vi "Motion Plot sub_VI.vi"(8 "Motion Parameters":T1={"Decel Time (s)"=0.0, "Accel Time (s)"=0.0, "Total Time (s)"=0.0, "Max Accel (mm/s^2)"=0.0, "Max Decel (mm/s^2)"=0.0, "Time step (s)"=0.01} {"Time step (s)" min=0.001}) -> (1 "Acceleration":dbl[](graph), 2 "Velocity":dbl[](graph), 3 "Displacement":dbl[](graph), 4 "V max (mm/s)":dbl, 5 "Dist max (mm)":dbl)   [LabVIEW 2017]
panel:
  # "Use 0.01s"
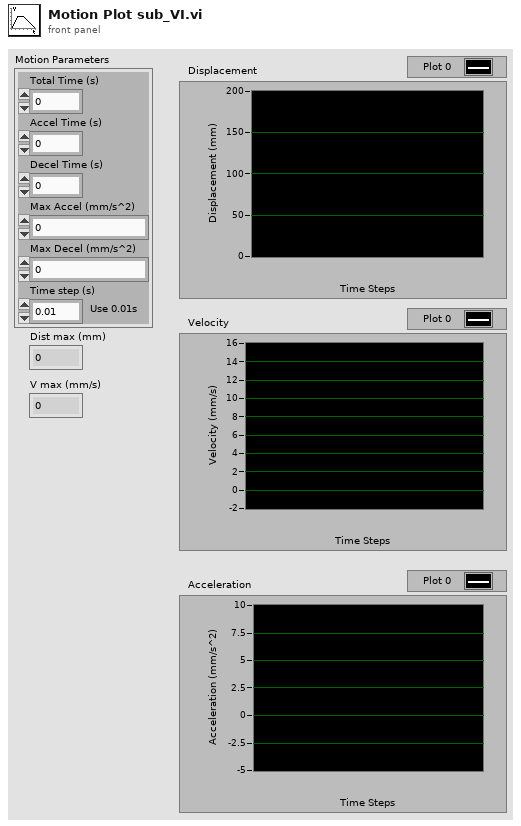
[diagram p1: front panel]
types:
  T1 = cluster{"Decel Time (s)":dbl, "Accel Time (s)":dbl, "Total Time (s)":dbl, "Max Accel (mm/s^2)":dbl, "Max Decel (mm/s^2)":dbl, "Time step (s)":dbl}
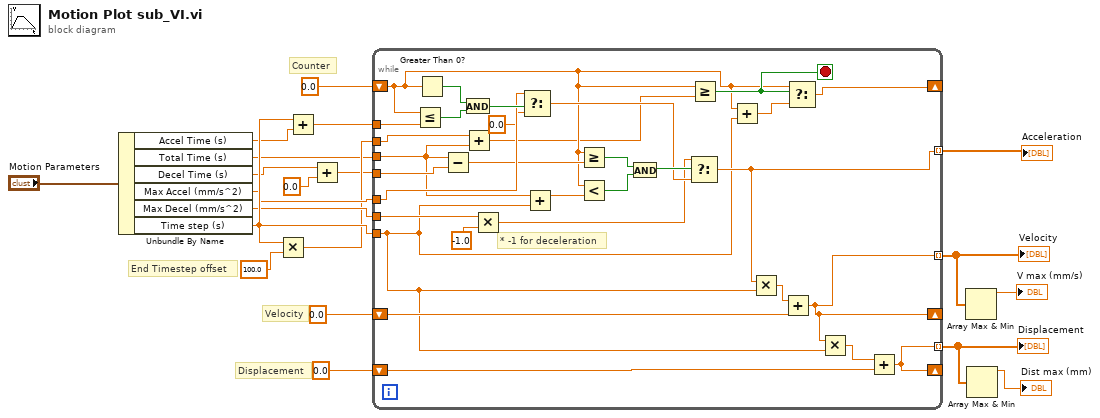
[diagram p0: block diagram]
diagram:
  # "End Timestep offset"
  # "Displacement"
  # "Velocity"
  # "Counter"
  n1 = Unbundle By Name("Motion Parameters") -> ("Accel Time (s)"=w3:dbl, "Total Time (s)"=w4:dbl, "Decel Time (s)"=w6:dbl, "Max Accel (mm/s^2)"=w16:dbl, "Max Decel (mm/s^2)"=w17:dbl, "Time step (s)"=w18:dbl)
  n2 = Multiply(x=w18, y=100.0) -> (x*y=w14:dbl)
  n3 = Add(x=w18, y=w3) -> (x+y=w10:dbl)
  n4 = Add(x=w6, y=0.0) -> (x+y=w11:dbl)
  n5 = while {
    shift-right: [w26] -> _
    shift-left: 0.0 -> [w25]
    tunnel: w10 -> [w51]
    tunnel: w16 -> [w47]
    tunnel: w4 -> [w39]
    tunnel: w11 -> [w44]
    tunnel: [w31] -> w5 mode=indexing
    tunnel: w17 -> [w28]
    shift-right: [w32] -> _
    shift-left: 0.0 -> [w36]
    shift-right: [w33] -> _
    shift-left: 0.0 -> [w34]
    tunnel: [w32] -> w19 mode=indexing
    tunnel: [w33] -> w2 mode=indexing
    tunnel: w18 -> [w23]
    tunnel: w14 -> [w21]
    stop <- w37 stop-if-true
    # "* -1 for deceleration"
    n6 = Less Or Equal?(x=w25, y=w51) -> (x <= y?=w49:bool)
    n7 = Greater Than 0?(x=w25) -> (x > 0?=w50:bool)
    n8 = Subtract(x=w39, y=w44) -> (x-y=w45:dbl)
    n9 = And(x=w50, y=w49) -> (x .and. y?=w48:bool)
    n10 = Add(x=w21, y=w39) -> (x+y=w22:dbl)
    n11 = Multiply(x=w28, y=-1.0 ("x")) -> (x*y=w29:dbl)
    n12 = Select(t=w47, s=w48, f=0.0) -> (s? t:f=w40:dbl)
    n13 = Add(x=w39, y=w23) -> (x+y=w24:dbl)
    n14 = Greater Or Equal?(x=w25, y=w45) -> (x >= y?=w43:bool)
    n15 = Less?(x=w25, y=w24) -> (x < y?=w42:bool)
    n16 = And(x=w43, y=w42) -> (x .and. y?=w41:bool)
    n17 = Select(t=w29, s=w41, f=w40) -> (s? t:f=w31:dbl)
    n18 = Greater Or Equal?(x=w25, y=w22) -> (x >= y?=w37:bool)
    n19 = Add(x=w25, y=w23) -> (x+y=w38:dbl)
    n20 = Multiply(x=w31, y=w23) -> (x*y=w35:dbl)
    n21 = Add(x=w35, y=w36) -> (x+y=w32:dbl)
    n22 = Select(t=w25, s=w37, f=w38) -> (s? t:f=w26:dbl)
    n23 = Multiply(x=w32, y=w23) -> (x*y=w30:dbl)
    n24 = Add(x=w30, y=w34) -> (x+y=w33:dbl)
  }
  "Acceleration" <- w5
  "Velocity" <- w19
  "Displacement" <- w2
  n25 = Array Max & Min(array=w19) -> (max value=→"V max (mm/s)":dbl)  [unwired: 3 out]
  n26 = Array Max & Min(array=w2) -> (max value=→"Dist max (mm)":dbl)  [unwired: 3 out]
